vi "Read_Write_Template.vi"(0 "Template File":path, 1 "Mode":T1, 5 "Channel names In":string[](array[string]), 7 "Single Value In":string, 9 "2D Info In":string[][](array[string]), 11 "1D Info In":string[](array[string]), 12 "Save file":bool=TRUE, 13 "Data type":string="Tolerance") -> (3 "Freshly Loaded?":bool, 4 "Template File Out":path, 6 "Template Ch Names Out":string[](array[string]), 8 "Single Value Out":string, 10 "2D Info Out":string[][](array[string]), 14 "Template Info":string[][](array[string]), 15 "1D Info Out":string[](array[string]))   [LabVIEW 2013]
uses:
  Controls/Global_mode.ctl
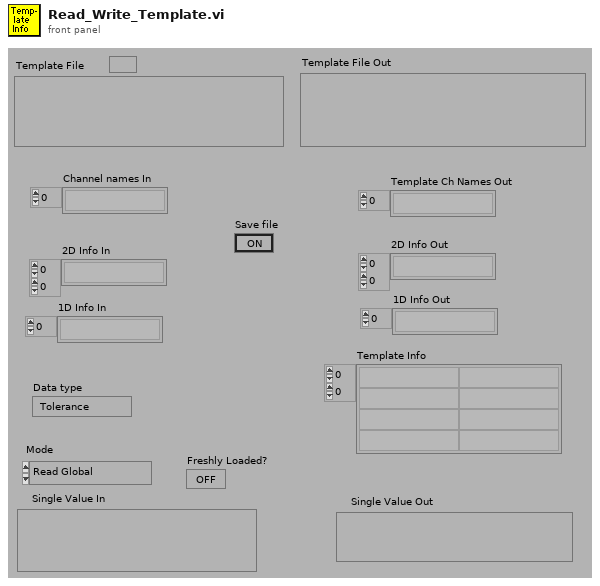
[diagram p1: front panel]
types:
  T1 = typedef "Global_mode.ctl" = enum16{"Read Global", "Load Global From File", "Write Global to File"}
  T2 = typedef "File_Status.ctl" = enum16{"Invalid Path", "This is a folder pathname", "Generic File Error", "Directory structure cannot be created", "File cannot be created", "File can be created", "File exist but read only", "File exist but no access", "File exist with read and write access"}
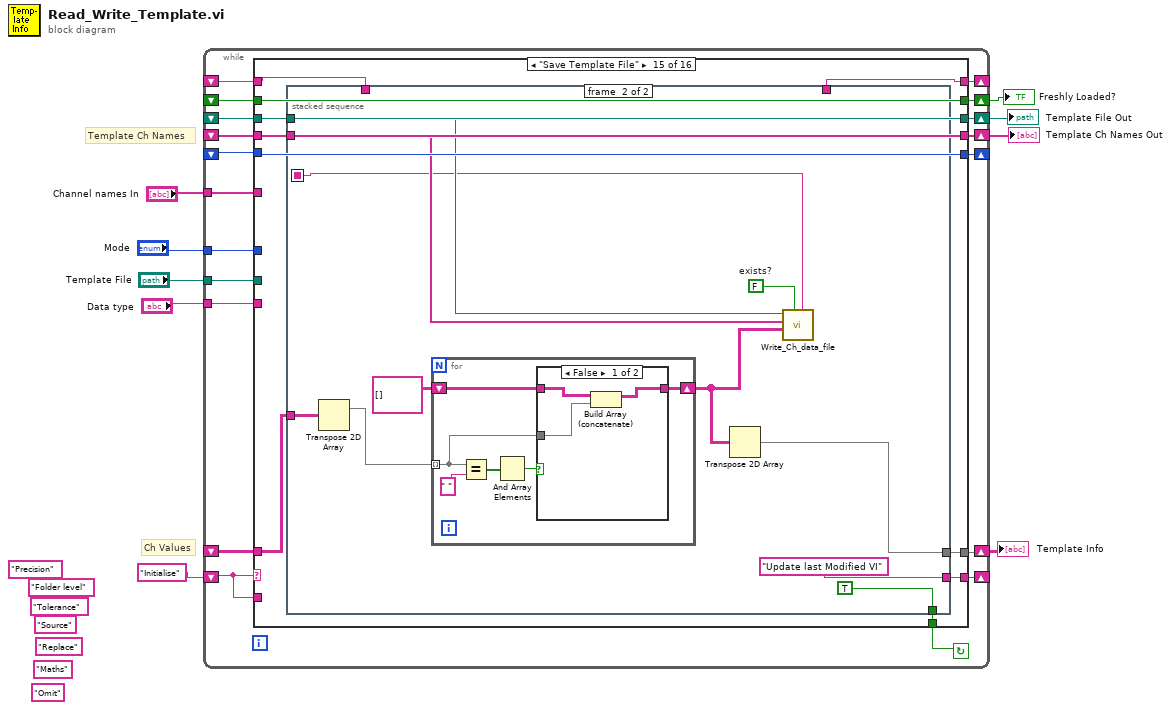
[diagram p0: block diagram]
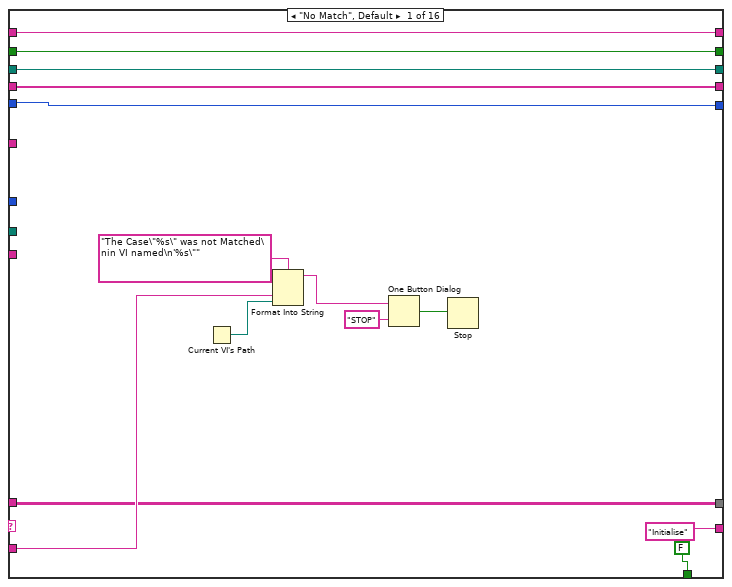
[diagram p2: hidden frame]
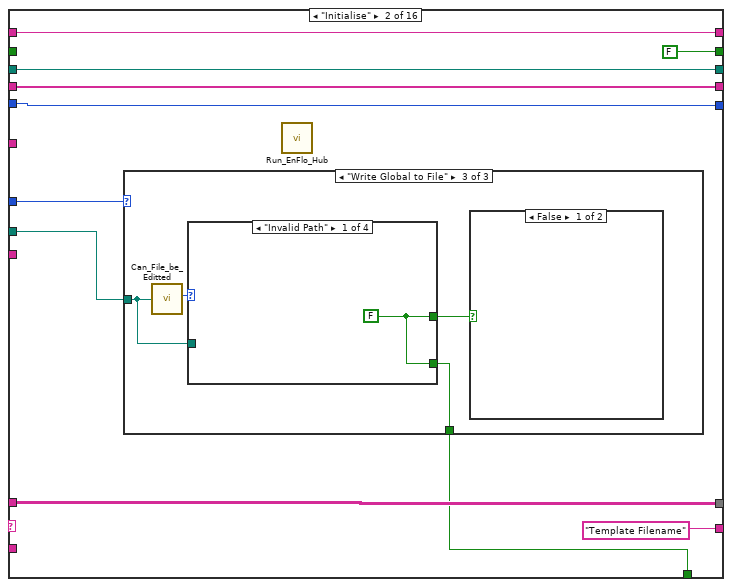
[diagram p3: hidden frame]
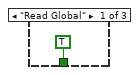
[diagram p4: hidden frame]
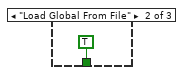
[diagram p5: hidden frame]
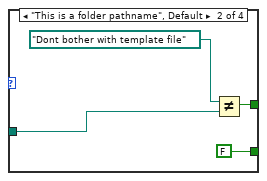
[diagram p6: hidden frame]
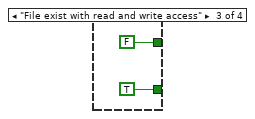
[diagram p7: hidden frame]
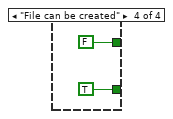
[diagram p8: hidden frame]
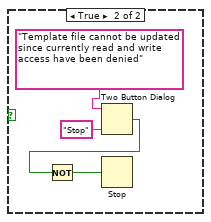
[diagram p9: hidden frame]
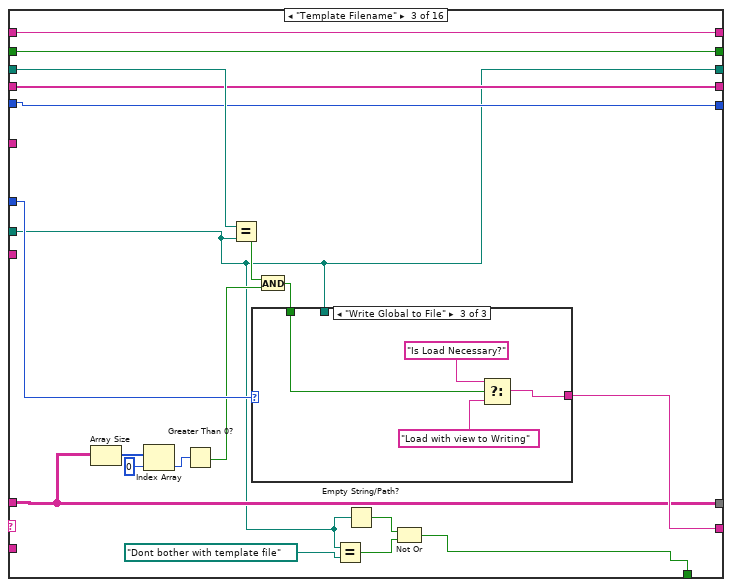
[diagram p10: hidden frame]
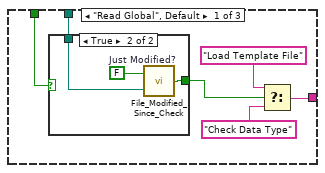
[diagram p11: hidden frame]
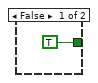
[diagram p12: hidden frame]
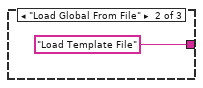
[diagram p13: hidden frame]
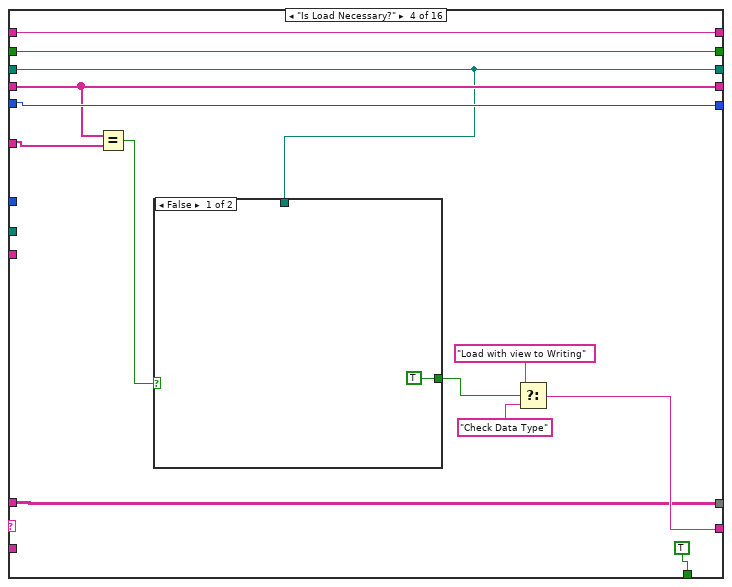
[diagram p14: hidden frame]
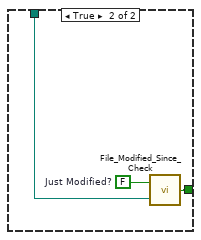
[diagram p15: hidden frame]
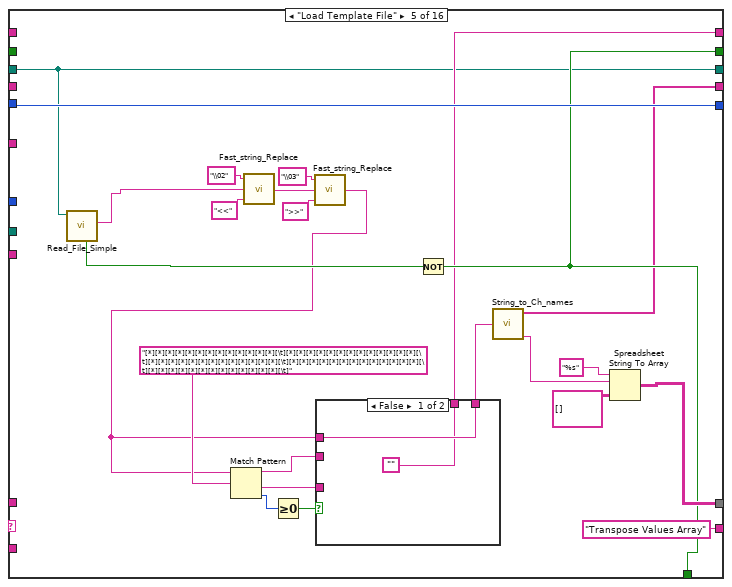
[diagram p16: hidden frame]
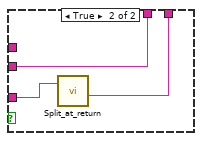
[diagram p17: hidden frame]
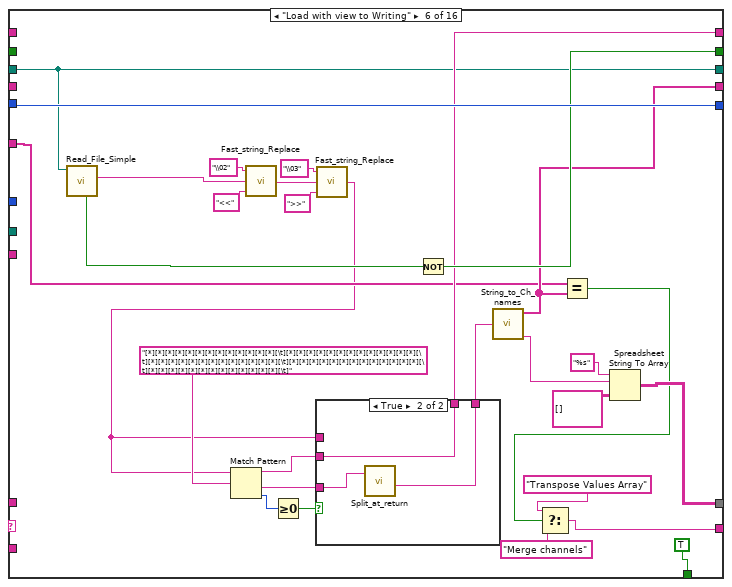
[diagram p18: hidden frame]
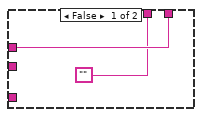
[diagram p19: hidden frame]
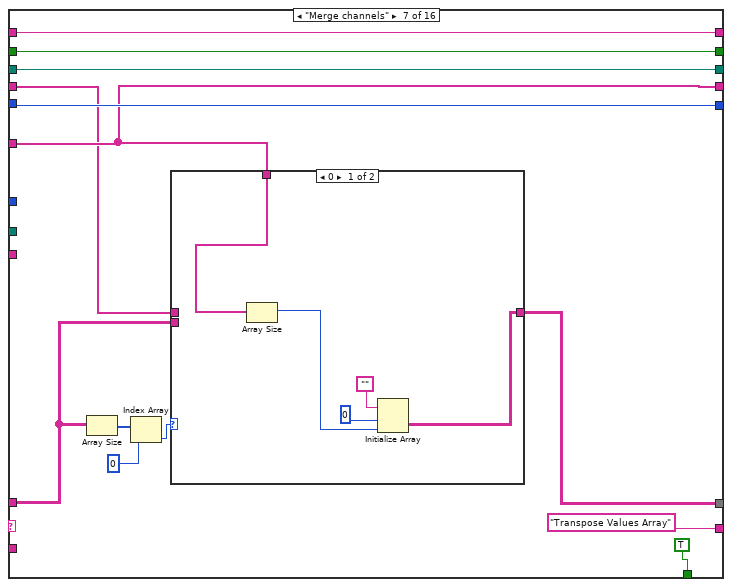
[diagram p20: hidden frame]
diagram:
  (unwired) "Precision"
  (unwired) "Folder level"
  (unwired) "Omit"
  (unwired) "Maths"
  (unwired) "Tolerance"
  (unwired) "Source"
  (unwired) "Replace"
  # "Template Ch Names"
  # "Ch Values"
  n1 = while {
    shift-left: _ -> [w13]
    shift-right: [w14] -> w2
    tunnel: "Channel names In" -> [w16]
    shift-left: _ -> [w15]
    shift-right: [w17] -> _
    tunnel: "Data type" -> [w18]
    shift-left: _ -> [w19]
    shift-right: [w20] -> w5
    shift-left: _ -> [w23]
    shift-right: [w22] -> w6
    shift-left: _ -> [w24]
    shift-right: [w25] -> w7
    tunnel: "Mode" -> [w26]
    shift-left: "Initialise" -> [w21]
    shift-right: [w27] -> _
    shift-right: [w12] -> _
    shift-left: _ -> [w11]
    tunnel: "Template File" -> [w10]
    stop <- w28 continue-if-true
    n2 = case shown="\"Save Template File\"" w21 {
      tunnel: [FALSE w43 w73 TRUE w139 TRUE ("Save file") TRUE ("Save file") TRUE w231 FALSE FALSE FALSE "Save file" FALSE ("Save file") w459 FALSE] -> w28
      tunnel: ["Initialise" "Template Filename" w87 w118 "Transpose Values Array" w162 "Transpose Values Array" "Check Data Type" w228 "" "" "" "Save Template File" "End" w456 "End"] -> w27
      tunnel: w26 -> [_ w45 w88 _ _ _ _ _ w230 _ _ _ _ _ _ _]
      tunnel: [w33 w51 w83 w112 w143 w178 w191 w218 w234 w298 w312 w332 w358 w445 w454 w504] -> w25
      tunnel: w24 -> [w33 w51 w83 w112 _ _ w189 w217 w234 w298 w312 w332 w359 w445 w453 w504]
      tunnel: w23 -> [w35 w52 w90 w108 w131 w159 w194 w213 w233 w300 w318 w334 w360 w439 w458 w503]
      tunnel: [w35 w52 w72 w108 w131 w159 w194 w213 w233 w300 w318 w334 w360 w439 w458 w503] -> w22
      tunnel: w21 -> [w37 _ _ _ _ _ _ _ _ _ _ _ _ _ _ _]
      tunnel: [w36 w50 w89 w111 w130 w166 w193 w212 w232 w296 w313 w329 w353 w448 w457 w502] -> w20
      tunnel: w19 -> [w36 w50 w89 w111 _ _ w192 w212 w232 w296 w313 w329 w353 w448 w457 w502]
      tunnel: w18 -> [_ _ _ _ _ _ _ _ w235 w299 w310 w333 w356 w441 _ _]
      tunnel: [w31 w48 w82 w116 w145 w180 w197 w211 w229 w289 w315 w321 w351 w447 w455 w500] -> w17
      tunnel: w16 -> [_ _ _ w110 _ w165 w193 _ _ w290 _ w326 w352 _ _ _]
      tunnel: w15 -> [w31 w48 w82 w116 w145 w180 w197 w211 _ w289 w315 w321 w351 w447 w455 w500]
      tunnel: [w30 FALSE w78 w107 w139 w174 w195 w209 w227 w288 w314 w320 w350 w446 w452 w498] -> w14
      tunnel: w13 -> [w30 _ w78 w107 _ _ w195 w209 w227 w288 w314 w320 w350 w446 w452 w498]
      tunnel: [w29 w46 w77 w106 w133 w168 w196 w208 w226 w287 w311 w319 w348 w443 w450 w497] -> w12
      tunnel: w11 -> [w29 w46 w77 w106 _ _ w196 w208 w226 w287 w311 w319 w348 w442 w451 w497]
      tunnel: w10 -> [_ w44 w72 _ _ _ _ _ _ _ _ _ _ _ _ _]
      frame "No Match", Default {
        n3 = Current VI's Path() -> (path=w38:path)
        n4 = Format Into String(format string="The Case\"%s\" was not Matched\nin VI named\n'%s\"" ("Format String"), w37, w38) -> (resulting string=w41:string)  [unwired: 2 in, 1 out]
        n5 = One Button Dialog(message=w41, button name ("OK")="STOP") -> (true=w39:bool)
        n6 = Stop(stop? (T)=w39) -> ()
      }
      frame "Initialise" {
        n7 = case shown="\"Write Global to File\"" w45 {
          tunnel: w44 -> [_ _ w55]
          tunnel: [TRUE TRUE w56] -> w43
          frame "Read Global" {
          }
          frame "Load Global From File" {
          }
          frame "Write Global to File" {
            n8 = call "Can_File_be_Editted.vi"("Filename"=w55) -> ("File Status"=w58:T2)  [unwired: 3 out]
            n9 = case shown="\"Invalid Path\"" w58 {
              tunnel: [w59 w61 FALSE FALSE] -> w57
              tunnel: [w59 FALSE TRUE TRUE] -> w56
              tunnel: w55 -> [_ w60 _ _]
              frame "Invalid Path" {
                w59 = FALSE
              }
              frame "This is a folder pathname", Default {
                n10 = Not Equal?(x=path "Dont bother with template file" ("Template File"), y=w60) -> (x != y?=w61:bool)
              }
              frame "File exist with read and write access" {
              }
              frame "File can be created" {
              }
            }
            n11 = case shown="False" w57 {
              frame False {
              }
              frame True {
                n12 = Two Button Dialog(message="Template file cannot be updated since currently read and write access have been denied", 1:"Stop" ("F button name (\"Cancel\")")) -> (T button?=w69:bool)  [unwired: 1 out]
                n13 = Not(x=w69) -> (.not. x?=w68:bool)
                n14 = Stop(stop? (T)=w68) -> ()
              }
            }
          }
        }
        n15 = call "Run_EnFlo_Hub.vi"() -> ()  [unwired: 8 out]
      }
      frame "Template Filename" {
        n16 = Array Size(array=w83) -> (size(s)=w84:i32[])
        n17 = Index Array(array=w84, index=0 ("Index")) -> (element=w86:i32)
        n18 = Greater Than 0?(x=w86) -> (x > 0?=w79:bool)
        n19 = Equal?(x=w90, y=w72) -> (x = y?=w81:bool)
        n20 = And(x=w81, y=w79) -> (x .and. y?=w80:bool)
        n21 = case shown="\"Write Global to File\"" w88 {
          tunnel: w80 -> [w96 _ w105]
          tunnel: [w92 "Load Template File" w103] -> w87
          tunnel: w72 -> [w95 _ _]
          frame "Read Global", Default {
            n22 = case shown="True" w96 {
              tunnel: w95 -> [_ w100]
              tunnel: [TRUE ("Modified?") w99] -> w94
              frame False {
              }
              frame True {
                w98 = FALSE  # Just Modified?
                n23 = call "File_Modified_Since_Check.vi"("Pathname"=w100, "Just Modified?"=w98) -> ("Modified?"=w99:bool)
              }
            }
            n24 = Select(t="Load Template File", s=w94, f="Check Data Type") -> (s? t:f=w92:string)
          }
          frame "Load Global From File" {
          }
          frame "Write Global to File" {
            n25 = Select(t="Is Load Necessary?", s=w105, f="Load with view to Writing") -> (s? t:f=w103:string)
          }
        }
        n26 = Equal?(x=w72, y=path "Dont bother with template file" ("Template File")) -> (x = y?=w75:bool)
        n27 = Empty String/Path?(string/path=w72) -> (empty?=w74:bool)
        n28 = Not Or(1:w75, 2:w74) -> (0:w73:bool)
      }
      frame "Is Load Necessary?" {
        n29 = Equal?(x=w111, y=w110) -> (x = y?=w109:bool)
        n30 = case shown="False" w109 {
          tunnel: w108 -> [_ w122]
          tunnel: [TRUE ("Modified?") w121] -> w115
          frame False {
          }
          frame True {
            w120 = FALSE  # Just Modified?
            n31 = call "File_Modified_Since_Check.vi"("Pathname"=w122, "Just Modified?"=w120) -> ("Modified?"=w121:bool)
          }
        }
        n32 = Select(t="Load with view to Writing", s=w115, f="Check Data Type") -> (s? t:f=w118:string)
      }
      frame "Load Template File" {
        n33 = call "Read_File_Simple.vi"("Filename"=w131) -> ("Error?"=w144:bool, "string"=w129:string)  [unwired: 2 in, 6 out]
        n34 = call "Fast_string_Replace.vi"("Replace match with:"="<<" ("regular expression"), "Input String"=w129, "regular expression"="\\02") -> ("Output String"=w123:string)  [unwired: 2 out]
        n35 = call "Fast_string_Replace.vi"("Replace match with:"=">>" ("regular expression"), "Input String"=w123, "regular expression"="\\03") -> ("Output String"=w128:string)  [unwired: 2 out]
        n36 = Match Pattern(string=w128, regular expression="[*][*][*][*][*][*][*][*][*][*][*][*][*][\t][*][*][*][*][*][*][*][*][*][*][*][*][*][\t][*][*][*][*][*][*][*][*][*][*][*][*][*][\t][*][*][*][*][*][*][*][*][*][*][*][*][*][\t][*][*][*][*][*][*][*][*][*][*][*][*][*][\t]" ("String")) -> (before substring=w132:string, after substring=w137:string, offset past match=w136:i32)  [unwired: 2 out]
        n37 = Greater Or Equal To 0?(x=w136) -> (x >= 0?=w135:bool)
        n38 = case shown="False" w135 {
          tunnel: w137 -> [_ w151]
          tunnel: [w148 w150] -> w134
          tunnel: w128 -> [w148 _]
          tunnel: ["" w149] -> w133
          tunnel: w132 -> [_ w149]
          frame False {
          }
          frame True {
            n39 = call "Split_at_return.vi"("String"=w151) -> ("after substring"=w150:string)  [unwired: 1 in, 3 out]
          }
        }
        n40 = Not(x=w144) -> (.not. x?=w139:bool)
        n41 = call "String_to_Ch_names.vi"("Spreadsheet string"=w134) -> ("Ch names"=w130:string[], "String After names"=w140:string)  [unwired: 2 out]
        n42 = Spreadsheet String To Array(format string="%s", spreadsheet string=w140, array type (2D Dbl)=string[][] [] ("Channel Values")) -> (array=w143:string[][])  [unwired: 1 out]
      }
      frame "Load with view to Writing" {
        n43 = call "Read_File_Simple.vi"("Filename"=w159) -> ("Error?"=w179:bool, "string"=w153:string)  [unwired: 2 in, 6 out]
        n44 = call "Fast_string_Replace.vi"("Replace match with:"="<<" ("regular expression"), "Input String"=w153, "regular expression"="\\02") -> ("Output String"=w154:string)  [unwired: 2 out]
        n45 = call "Fast_string_Replace.vi"("Replace match with:"=">>" ("regular expression"), "Input String"=w154, "regular expression"="\\03") -> ("Output String"=w152:string)  [unwired: 2 out]
        n46 = Match Pattern(string=w152, regular expression="[*][*][*][*][*][*][*][*][*][*][*][*][*][\t][*][*][*][*][*][*][*][*][*][*][*][*][*][\t][*][*][*][*][*][*][*][*][*][*][*][*][*][\t][*][*][*][*][*][*][*][*][*][*][*][*][*][\t][*][*][*][*][*][*][*][*][*][*][*][*][*][\t]" ("String")) -> (before substring=w167:string, after substring=w172:string, offset past match=w171:i32)  [unwired: 2 out]
        n47 = Greater Or Equal To 0?(x=w171) -> (x >= 0?=w170:bool)
        n48 = case shown="True" w170 {
          tunnel: w172 -> [_ w185]
          tunnel: [w182 w184] -> w169
          tunnel: w152 -> [w182 _]
          tunnel: ["" w183] -> w168
          tunnel: w167 -> [_ w183]
          frame False {
          }
          frame True {
            n49 = call "Split_at_return.vi"("String"=w185) -> ("after substring"=w184:string)  [unwired: 1 in, 3 out]
          }
        }
        n50 = Not(x=w179) -> (.not. x?=w174:bool)
        n51 = call "String_to_Ch_names.vi"("Spreadsheet string"=w169) -> ("Ch names"=w166:string[], "String After names"=w175:string)  [unwired: 2 out]
        n52 = Equal?(x=w165, y=w166) -> (x = y?=w164:bool)
        n53 = Select(t="Transpose Values Array", s=w164, f="Merge channels") -> (s? t:f=w162:string)
        n54 = Spreadsheet String To Array(format string="%s", spreadsheet string=w175, array type (2D Dbl)=string[][] [] ("Channel Values")) -> (array=w178:string[][])  [unwired: 1 out]
      }
      frame "Merge channels" {
        n55 = Array Size(array=w189) -> (size(s)=w188:i32[])
        n56 = Index Array(array=w188, index=0) -> (element=w186:i32)
        n57 = case shown="0" w186 {
          tunnel: w193 -> [w200 w207]
          tunnel: w192 -> [_ w206]
          tunnel: w189 -> [_ w205]
          tunnel: [w199 w204] -> w191
          frame 0 {
            n58 = Array Size(array=w200) -> (size(s)=w201:i32)
            n59 = Initialize Array("", 0 ("Dimension Size"), w201) -> (w199:string[][])
          }
          frame 1, Default {
            n60 = call "Merge_2D_values.vi"("Values In"=w205, "Present Channels"=w206, "Desired Channels"=w207) -> ("Values Out"=w204:string[][])
          }
        }
      }
      frame "Transpose Values Array" {
        n61 = Array Size(array=w217) -> (size(s)=w215:i32[])
        n62 = Index Array(array=w215, index=1 ("Index")) -> (element=w214:i32)
        n63 = for {
          N: w214 -> [_]
          tunnel: w217 -> [w222]
          tunnel: [w223] -> w218 mode=indexing
          i -> [w221]
          n64 = Index Array(array=w222, index (col)=w221) -> (element=w220:string[])  [unwired: 1 in]
          n65 = for {
            tunnel: [w225] -> w223 mode=indexing
            tunnel: w220 -> [w224] mode=indexing
            n66 = call "Remove_Quotes.vi"("String"=w224) -> ("String Out"=w225:string)
          }
        }
      }
      frame "Check Data Type" {
        n67 = case shown="\"Ignore When\"" w235 {
          tunnel: [1 1 1 1 1 2 1 1 2 2 2 1 2 1 1 0] -> w229
          tunnel: w235 -> [w246 _ _ _ _ _ _ _ _ _ _ _ _ _ _ _]
          tunnel: [w245 TRUE TRUE TRUE TRUE TRUE TRUE TRUE TRUE TRUE TRUE TRUE TRUE TRUE TRUE TRUE] -> w231
          frame "No Match", Default {
            n68 = Empty String/Path?(string/path=w246) -> (empty?=w247:bool)
            n69 = case shown="False" w247 {
              tunnel: w246 -> [w250 _]
              tunnel: [FALSE FALSE] -> w245
              frame False {
                n70 = Current VI's Path() -> (path=w251:path)
                n71 = Format Into String(format string="The Case\"%s\" was not Matched\nin VI named\n'%s\"" ("Format String"), w250, w251) -> (resulting string=w254:string)  [unwired: 2 in, 1 out]
                n72 = One Button Dialog(message=w254, button name ("OK")="STOP") -> (true=w252:bool)
                n73 = Stop(stop? (T)=w252) -> ()
              }
              frame True {
              }
            }
          }
          frame "Description" {
          }
          frame "Dispose" {
          }
          frame "Decimal" {
          }
          frame "Precision" {
          }
          frame "Multiple Sources" {
          }
          frame "Summarise" {
          }
          frame "Tolerance" {
          }
          frame "Source" {
          }
          frame "Replace" {
          }
          frame "Ignore When" {
          }
          frame "Maths" {
          }
          frame "Omit" {
          }
          frame "Folder level" {
          }
          frame "Minimum Value" {
          }
          frame "Log Folder Name" {
          }
        }
        n74 = case shown="\"Write Global to File\"" w230 {
          tunnel: w229 -> [w237 w241]
          tunnel: [w236 w242] -> w228
          frame "Read Global", Default {
            n75 = case shown="0" w237 {
              tunnel: ["Create Outputs 2D" "Create Outputs 1D" "Create single value output"] -> w236
              frame 2, Default {
              }
              frame 1 {
              }
              frame 0 {
              }
            }
          }
          frame "Write Global to File" {
            n76 = case shown="1, Default" w241 {
              tunnel: ["Replace single value" "Replace Values"] -> w242
              frame 0 {
              }
              frame 1, Default {
              }
            }
          }
        }
      }
      frame "Create Outputs 1D" {
        n77 = for {
          tunnel: w299 -> [w308]
          tunnel: w298 -> [w307] mode=indexing
          tunnel: [w306] -> w297 mode=indexing
          n78 = call "Get_Array_Subset.vi"("String Array In"=w307, "Subset Name"=w308) -> ("First Element"=w306:string)  [unwired: 4 out]
        }
        n79 = Array Size(array=w290) -> (size(s)=w292:i32)
        n80 = Equal To 0?(x=w292) -> (x = 0?=w291:bool)
        n81 = case shown="False" w291 {
          tunnel: w297 -> [w304 w305]
          tunnel: w290 -> [w303 _]
          tunnel: w296 -> [w302 _]
          tunnel: [w301 w305] -> w295
          frame False {
            n82 = call "Merge_row_values.vi"("Present Row values"=w304, "Present Channels"=w302, "Desired Channels"=w303) -> ("Desired Row values"=w301:string[])  [unwired: 1 out]
          }
          frame True {
          }
        }
        "1D Info Out" <- w295
      }
      frame "Create single value output" {
        n83 = call "Get_Characters_from_string.vi"("Input string"=w311, "Variable name"=w310) -> ("Value"=→"Single Value Out":string)  [unwired: 1 in, 1 out]
      }
      frame "Create Outputs 2D" {
        n84 = for {
          tunnel: w333 -> [w347]
          tunnel: w332 -> [w346] mode=indexing
          tunnel: [w345] -> w328 mode=indexing
          n85 = call "Get_Array_Subset.vi"("String Array In"=w346, "Subset Name"=w347) -> ("Array Subset Out"=w345:string[])  [unwired: 4 out]
        }
        n86 = Equal?(x=w329, y=w326) -> (x = y?=w324:bool)
        n87 = Array Size(array=w326) -> (size(s)=w325:i32)
        n88 = Equal To 0?(x=w325) -> (x = 0?=w323:bool)
        n89 = Or(x=w324, y=w323) -> (x .or. y?=w322:bool)
        n90 = case shown="False" w322 {
          tunnel: w329 -> [w338 _]
          tunnel: w326 -> [w337 _]
          tunnel: w328 -> [w336 w344]
          tunnel: [w335 w344] -> w327
          frame False {
            n91 = for {
              tunnel: w338 -> [w343]
              tunnel: w337 -> [w342] mode=indexing
              tunnel: w336 -> [w340]
              tunnel: [w339] -> w335 mode=indexing
              n92 = Search 1D Array(1D array=w343, element=w342) -> (index of element=w341:i32)  [unwired: 1 out]
              n93 = Index Array(array=w340, index (row)=w341) -> (element=w339:string[])  [unwired: 1 in]
            }
          }
          frame True {
          }
        }
        "2D Info Out" <- w327
      }
      frame "Replace Values" {
        n94 = for {
          tunnel: w356 -> [w369]
          tunnel: w359 -> [w368] mode=indexing
          tunnel: [w367] -> w358 mode=indexing
          tunnel: w353 -> [w366] mode=indexing
          tunnel: w351 -> [w365]
          tunnel: "1D Info In" -> [w364]
          tunnel: "2D Info In" -> [w363]
          tunnel: w353 -> [w362] mode=indexing
          tunnel: w352 -> [w361]
          n95 = stacked-sequence {
            seq-local: [_ w379 _ _ _] -> [_ _ _ w430 _]
            seq-local: [_ w378 _ _ _] -> [_ _ _ w431 _]
            seq-local: [_ _ w390 _ _] -> [_ _ _ w429 _]
            seq-local: [_ w377 _ _ _] -> [_ _ w386 _ _]
            seq-local: [w372 _ _ _ _] -> [_ _ w387 _ _]
            seq-local: [w370 _ _ _ _] -> [_ _ w385 _ _]
            tunnel: w369 -> [_ w384 _ w432 _]
            tunnel: w368 -> [_ w381 _ _ _]
            tunnel: [_ _ _ w422 _] -> w367
            tunnel: w366 -> [_ _ _ w423 _]
            tunnel: w365 -> [w371 _ _ _ _]
            tunnel: w364 -> [_ _ w389 _ _]
            tunnel: w363 -> [_ _ w388 _ _]
            tunnel: w362 -> [w374 _ _ _ _]
            tunnel: w361 -> [w373 _ _ _ _]
            frame #0 {
              n96 = Search 1D Array(1D array=w373, element=w374) -> (index of element=w370:i32)  [unwired: 1 out]
              n97 = case shown="0, Default" w370 {
                tunnel: [w375 0] -> w372
                tunnel: w371 -> [w375 _]
                frame 0, Default {
                }
                frame -1 {
                }
              }
            }
            frame #1 {
              n98 = call "Get_Array_Subset.vi"("String Array In"=w381, "Subset Name"=w384) -> ("index after match"=w380:i32, "Array Subset Out"=w377:string[], "Length before match"=w382:i32)  [unwired: 2 out]
              n99 = Array Subset(array=w381, index=0 ("Array Index"), length=w382) -> (w379:string[])
              n100 = Array Subset(array=w381, index=w380) -> (w378:string[])  [unwired: 1 in]
            }
            frame #2 {
              n101 = case shown="2, Default" w387 {
                tunnel: [w394 w418 w421] -> w390
                tunnel: w389 -> [_ w420 _]
                tunnel: w388 -> [w393 _ _]
                tunnel: w386 -> [_ _ w421]
                tunnel: w385 -> [w391 w417 _]
                frame 2, Default {
                  n102 = Index Array(array=w393, index (row)=w391) -> (element=w392:string[])  [unwired: 1 in]
                  n103 = while {
                    shift-left: _ -> [w395]
                    shift-right: [w396] -> _
                    tunnel: [w397] -> w394
                    tunnel: w392 -> [w399]
                    i -> [w400]
                    stop <- w398 continue-if-true
                    n104 = case shown="0, Default" w400 {
                      tunnel: w399 -> [w402 w405]
                      tunnel: [w403 FALSE] -> w398
                      tunnel: [w402 w408] -> w397
                      tunnel: [w401 w407] -> w396
                      tunnel: w395 -> [_ w407]
                      frame 0, Default {
                        n105 = Empty String/Path?(string/path=w402) -> (empty?=w401:bool[])
                        n106 = Or Array Elements(Boolean array=w401) -> (logical OR=w403:bool)
                      }
                      frame 1 {
                        n107 = for {
                          shift-right: [w411] -> w408
                          shift-left: string[] [] -> [w410]
                          tunnel: w407 -> [w412] mode=indexing
                          tunnel: w405 -> [w409] mode=indexing
                          n108 = case shown="True" w412 {
                            tunnel: [w414 w416] -> w411
                            tunnel: w410 -> [w415 w416]
                            tunnel: w409 -> [w413 _]
                            frame False {
                              n109 = Build Array (concatenate)(w415, w413) -> (w414:string[])
                            }
                            frame True {
                            }
                          }
                        }
                      }
                    }
                  }
                }
                frame 1 {
                  n110 = Index Array(array=w420, index=w417) -> (element=w419:string)
                  n111 = Build Array(w419) -> (w418:string[])
                }
                frame 0 {
                }
              }
            }
            frame #3 {
              w424 = ""
              n112 = Format Into String(format string="**%s Start**" ("Format String"), w432) -> (resulting string=w428:string)  [unwired: 2 in, 1 out]
              n113 = Format Into String(format string="**%s End**" ("Format String"), w432) -> (resulting string=w427:string)  [unwired: 2 in, 1 out]
              n114 = Build Array (concatenate)(w430, w428, w429, w427, w431) -> (w426:string[])
              n115 = call "Clean_Up_Template.vi"("Template Info In"=w426) -> ("Template Info Out"=w425:string[])
              n116 = Build Array (concatenate)(w424, w423, w424, w425) -> (w422:string[])
            }
            frame #4 {
            }
          }
        }
      }
      frame "Replace single value" {
        w436 = FALSE  # append to file? (new file:F)
        w437 = FALSE  # advisory dialog? (display:T)
        n117 = call "Read_File_Simple.vi"("Filename"=w439) -> ("string"=w440:string)  [unwired: 2 in, 7 out]
        n118 = call "Replace_data_in_setup_string.vi"("New data string"="Single Value In", "Input string"=w442, "Variable name"=w441) -> ("Appended string"=w443:string)
        n119 = call "Replace_data_in_setup_string.vi"("New data string"="Single Value In", "Input string"=w440, "Variable name"=w441) -> ("Appended string"=w438:string)
        n120 = call "Write_Characters_To_File.vi"("file path (dialog if empty)"=w439, "advisory dialog? (display:T)"=w437, "character string"=w438, "append to file? (new file:F)"=w436) -> ()  [unwired: 1 in, 4 out]
      }
      frame "Save Template File" {
        n121 = stacked-sequence {
          seq-local: [w462 _] -> [_ w476]
          tunnel: [_ TRUE] -> w459
          tunnel: w458 -> [_ w486]
          tunnel: w457 -> [_ w485]
          tunnel: [_ "Update last Modified VI"] -> w456
          tunnel: [_ w479] -> w454
          tunnel: w453 -> [_ w478]
          tunnel: w451 -> [w461 _]
          tunnel: [w460 _] -> w450
          frame #0 {
            w467 = "Log Folder Name" ("Variable name")
            n122 = call "Get_Characters_from_string.vi"("Input string"=w461, "Variable name"=w467) -> ("Status"=w468:enum16{"Char in string", "Char not in string"})  [unwired: 1 in, 1 out]
            n123 = case shown="\"Char not in string\"" w468 {
              tunnel: w467 -> [_ w475]
              tunnel: w461 -> [w469 w471]
              tunnel: [w469 w470] -> w460
              frame "Char in string" {
              }
              frame "Char not in string" {
                n124 = Default Directory() -> (w474:path)
                n125 = Path To String(path=w474) -> (string=w473:string)
                n126 = call "Characters_to_string.vi"("Characters to write"=w473, "Label for characters"=w475) -> ("Output string"=w472:string)
                n127 = Concatenate Strings(w471, w472) -> (w470:string)
              }
            }
            n128 = Initialize Array("", 10 ("Dimension Size")) -> (w466:string[])
            n129 = call "Asterisk_header.vi"("Channel names"=w466) -> ("Header string"=w463:string)
            n130 = Concatenate Strings(w460, w463) -> (w462:string)
          }
          frame #1 {
            w484 = FALSE  # exists?
            n131 = Transpose 2D Array(2D array=w478) -> (transposed array=w482:string[][])
            n132 = for {
              shift-right: [w489] -> w480
              shift-left: string[][] [] -> [w488]
              tunnel: w482 -> [w487] mode=indexing
              n133 = Equal?(x=w487, y=" ") -> (x = y?=w491:bool[])
              n134 = And Array Elements(Boolean array=w491) -> (logical AND=w490:bool)
              n135 = case shown="False" w490 {
                tunnel: [w494 w496] -> w489
                tunnel: w488 -> [w495 w496]
                tunnel: w487 -> [w493 _]
                frame False {
                  n136 = Build Array (concatenate)(w495, w493) -> (w494:string[][])
                }
                frame True {
                }
              }
            }
            n137 = Transpose 2D Array(2D array=w480) -> (transposed array=w479:string[][])
            n138 = call "Write_Ch_data_file.vi"("Header string"=w476, "exists?"=w484, "Channel Values"=w480, "Channel names"=w485, "Filename"=w486) -> ()  [unwired: 3 in, 4 out]
          }
        }
      }
      frame "Update last Modified VI" {
        w499 = TRUE  # Just Modified?
        n139 = call "File_Modified_Since_Check.vi"("Pathname"=w503, "Just Modified?"=w499) -> ()  [unwired: 1 out]
      }
    }
  }
  "Template Ch Names Out" <- w5
  "Template File Out" <- w6
  "Template Info" <- w7
  "Freshly Loaded?" <- w2
